vi "Min_max_average.vi"() -> ()   [LabVIEW 2025]
panel:
  out "Oven's Temperature":cluster{dbl, dbl, dbl}(slide)={0.0, 6.848874598070739, 5.434083601286173} scale=175.0..280.0
  out "min value":dbl
  out "max value":dbl
  out "Mean value":dbl
  out "size(s)":i32
  in  "File Path":path
  in  "?":bool
  in  "Choose oven":dbl
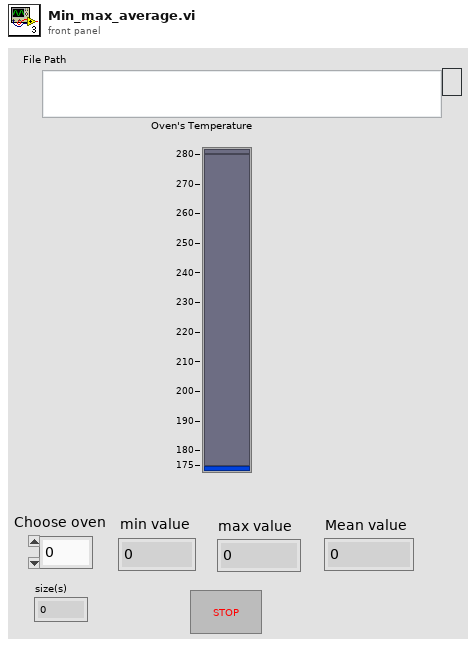
[diagram p1: front panel]
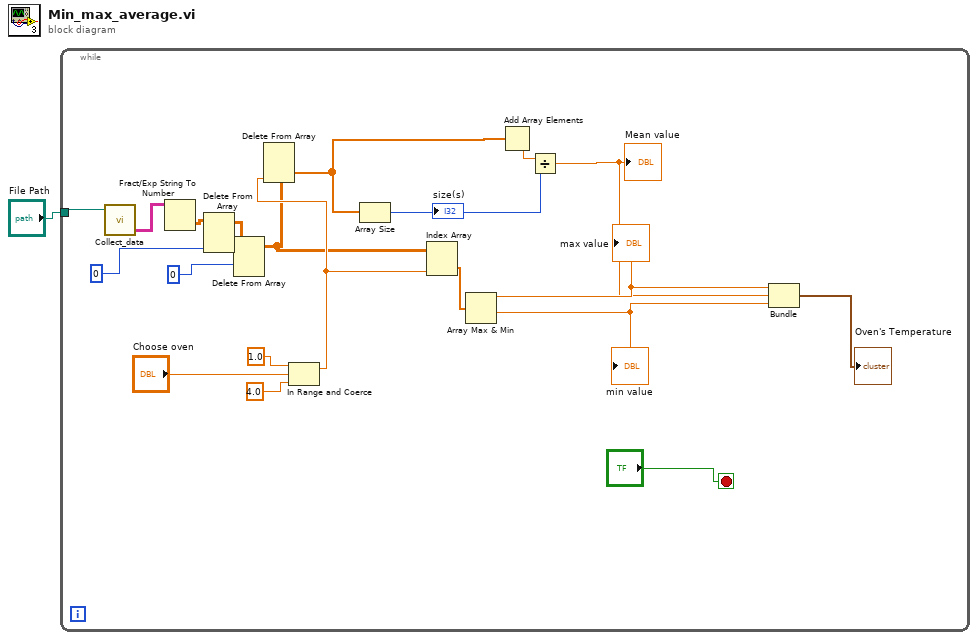
[diagram p0: block diagram]
diagram:
  n1 = while {
    tunnel: "File Path" -> [w20]
    stop <- "?" stop-if-true
    n2 = call "Collect_data.vi"("File Path"=w20) -> ("all rows"=w13:string[][])  [unwired: 1 in]
    n3 = Fract/Exp String To Number(string=w13) -> (number=w6:dbl[][])  [unwired: 3 in, 1 out]
    n4 = Delete From Array(array=w6, index (col)=0 ("disabled index (col)")) -> (array with subset deleted=w8:dbl[][])  [unwired: 2 in, 1 out]
    n5 = Delete From Array(array=w8, index (row)=0) -> (array with subset deleted=w7:dbl[][])  [unwired: 2 in, 1 out]
    n6 = In Range and Coerce(upper limit=1.0, x="Choose oven", lower limit=4.0) -> (coerced(x)=w16:dbl)  [unwired: 1 out]
    n7 = Delete From Array "Delete From Array"(array=w7, index (col)=w16) -> (deleted portion=w12:dbl[])  [unwired: 2 in, 1 out]
    n8 = Array Size(array=w12) -> (size(s)=w14:i32)
    "size(s)" <- w14
    n9 = Index Array "Index Array"(array=w7, index (col)=w16) -> (element=w10:dbl[])  [unwired: 1 in]
    n10 = Array Max & Min(array=w10) -> (max value=w5:dbl, min value=w3:dbl)  [unwired: 2 out]
    "max value" <- w5
    "min value" <- w3
    n11 = Add Array Elements(numeric array=w12) -> (sum=w15:dbl)
    n12 = Divide(x=w15, y=w14) -> (x/y=w4:dbl)
    "Mean value" <- w4
    n13 = Bundle(w5, w4, w3) -> (→"Oven's Temperature":cluster{dbl, dbl, dbl})  [unwired: 1 in]
  }
